vi "Create Event Reader.vi"(8 "error in (no error)":errorcluster, 11 "Enclave in":refnum<class "Enclave.lvclass">) -> (0 "error out":errorcluster, 2 "Event":refnum<class "Event.lvclass">, 3 "Enclave out":refnum<class "Enclave.lvclass">)   [LabVIEW 2022 SP3, in "Enclave.lvlib" / "Enclave.lvclass"]
uses:
  Enclave.lvclass
  Event/Event.lvclass
  Enclave.lvclass/Enclave.ctl
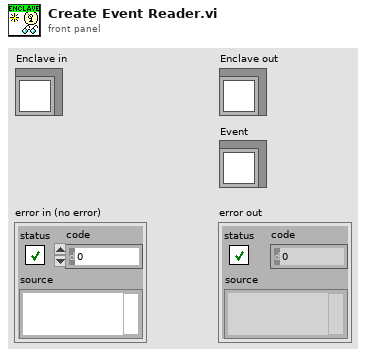
[diagram p1: front panel]
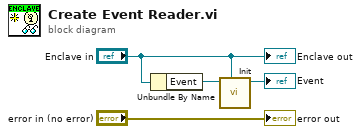
[diagram p0: block diagram]
diagram:
  n1 = Unbundle By Name("Enclave in") -> ("Event"=w1:refnum<user-event>)
  n2 = call "Init.vi"("Enclave"="Enclave in", "Event"=w1) -> ("Event out"=→"Event":refnum<class "Event.lvclass">)  [unwired: 8 in, 1 out]
  "error out" <- "error in (no error)"
  "Enclave out" <- "Enclave in"
